vi "Change mode.vi"(10 "Set Mode":T1=enum."Realtime mode") -> (0 "Prev Mode":T1=enum."Realtime mode", 3 "Current Mode":T1=enum."Realtime mode")   [LabVIEW 2020]
uses:
  Typedef/Mode.ctl
  Global variable.vi
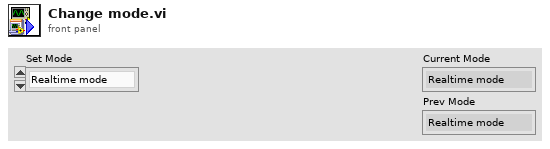
[diagram p1: front panel]
types:
  T1 = typedef "Mode.ctl" = enum16{"Schedule mode", "Manual mode", "Realtime mode", ""}
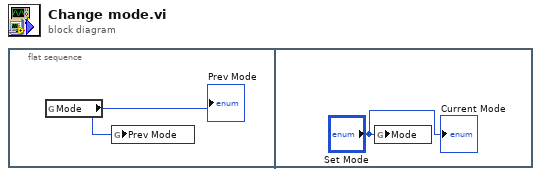
[diagram p0: block diagram]
diagram:
  n1 = flat-sequence {
    frame #0 {
      n2 = global read "Global variable.vi" "Mode"() -> (w1:T1)
      "Prev Mode" <- w1
      n3 = global write "Global variable.vi" "Prev Mode"(w1) -> ()
    }
    frame #1 {
      n4 = global write "Global variable.vi" "Mode"("Set Mode") -> ()
      "Current Mode" <- "Set Mode"
    }
  }
